vi "getMeasurement.vi"(7 "Source":string, 8 "error in (no error)":errorcluster, 10 "Measurement":T1=enum."Voltage Peak-Peak", 11 "ScopeKeysight in":refnum<class "ScopeKeysight.lvclass">) -> (0 "error out":errorcluster, 2 "Result":dbl, 3 "ScopeKeysight out":refnum<class "ScopeKeysight.lvclass">)   [LabVIEW 2023, in "ScopeKeysight.lvclass"]
doc: "<b>Author:</b> Wolfgang\n<b>Description:</b> returns a measurement"
uses:
  ScopeKeysight.lvclass
  Data/scopeMeasurements.ctl
  ScopeKeysight.lvclass/ScopeKeysight.ctl
  Driver/Public/Data/Read Measurement (Current Value).vi
  Driver/Keysight-DSQx3014T.lvlib
  sweScope.lvlib
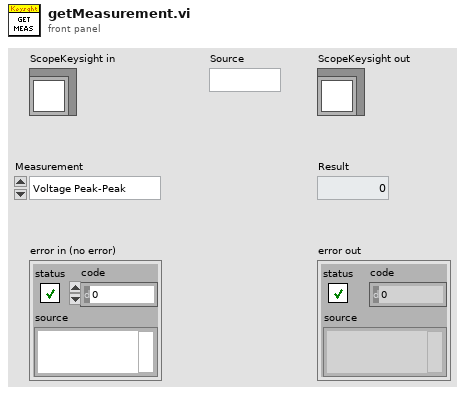
[diagram p1: front panel]
types:
  T1 = typedef "sweScope.lvlib/scopeMeasurements.ctl" = enum16{"Disable", "Mean", "Voltage Peak-Peak", "Frequency", "Amplitude", "Period", "Falling Slew Rate", "Rising Slew Rate"}
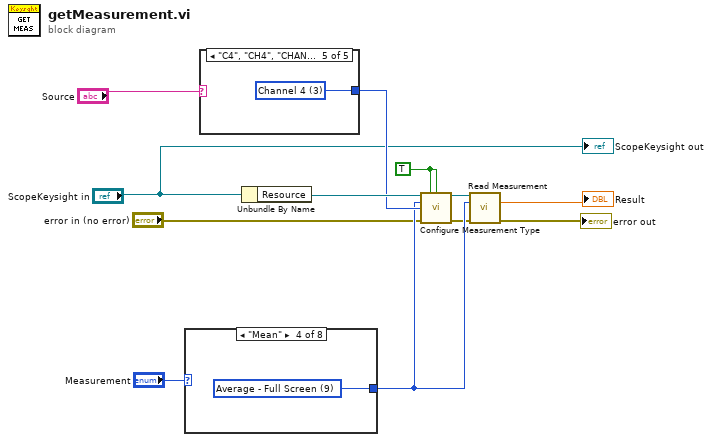
[diagram p0: block diagram]
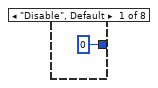
[diagram p2: hidden frame]
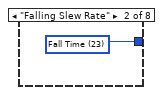
[diagram p3: hidden frame]
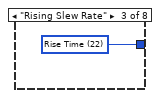
[diagram p4: hidden frame]
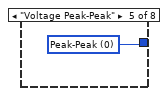
[diagram p5: hidden frame]
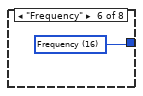
[diagram p6: hidden frame]
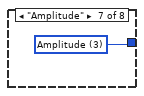
[diagram p7: hidden frame]
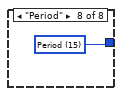
[diagram p8: hidden frame]
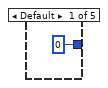
[diagram p9: hidden frame]
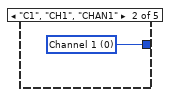
[diagram p10: hidden frame]
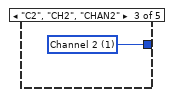
[diagram p11: hidden frame]
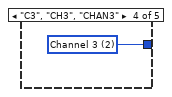
[diagram p12: hidden frame]
diagram:
  w1 = TRUE ("Enable Clear (F: Disable)")
  n1 = case shown="\"Mean\"" "Measurement" {
    tunnel: [0 ("Measurement Type (0: Peak-Peak)") w14 w15 w16 w17 w18 w19 w20] -> w8
    frame "Disable", Default {
    }
    frame "Falling Slew Rate" {
      w14 = 23 items=["Peak-Peak", "Maximum", "Mimimum", "Amplitude", "Top", "Base", "Overshoot", "Preshoot", "Average - N Cycles", "Average - Full Screen", "DC RMS - N Cycles", "DC RMS - Full Screen", "AC RMS - N Cycles", "AC RMS - Full Screen (Std Dev)", "Ratio", "Period", "Frequency", "Counter", "+Width", "-Width", "Burst Width", "Duty Cycle", "Rise Time", "Fall Time", "Delay", "Phase", "X minY", "X maxY", "Positive Pulse Count", "Negative Pulse Count", "Raising Edge Count", "Falling Edge Count", "Area - N Cycle", "Area - Full Screen", "Bit Rate", "Negtive Duty Cycle", "Standard Deviation"] ("Measurement Type (0: Peak-Peak)")
    }
    frame "Rising Slew Rate" {
      w15 = 22 items=["Peak-Peak", "Maximum", "Mimimum", "Amplitude", "Top", "Base", "Overshoot", "Preshoot", "Average - N Cycles", "Average - Full Screen", "DC RMS - N Cycles", "DC RMS - Full Screen", "AC RMS - N Cycles", "AC RMS - Full Screen (Std Dev)", "Ratio", "Period", "Frequency", "Counter", "+Width", "-Width", "Burst Width", "Duty Cycle", "Rise Time", "Fall Time", "Delay", "Phase", "X minY", "X maxY", "Positive Pulse Count", "Negative Pulse Count", "Raising Edge Count", "Falling Edge Count", "Area - N Cycle", "Area - Full Screen", "Bit Rate", "Negtive Duty Cycle", "Standard Deviation"] ("Measurement Type (0: Peak-Peak)")
    }
    frame "Mean" {
      w16 = 9 items=["Peak-Peak", "Maximum", "Mimimum", "Amplitude", "Top", "Base", "Overshoot", "Preshoot", "Average - N Cycles", "Average - Full Screen", "DC RMS - N Cycles", "DC RMS - Full Screen", "AC RMS - N Cycles", "AC RMS - Full Screen (Std Dev)", "Ratio", "Period", "Frequency", "Counter", "+Width", "-Width", "Burst Width", "Duty Cycle", "Rise Time", "Fall Time", "Delay", "Phase", "X minY", "X maxY", "Positive Pulse Count", "Negative Pulse Count", "Raising Edge Count", "Falling Edge Count", "Area - N Cycle", "Area - Full Screen", "Bit Rate", "Negtive Duty Cycle", "Standard Deviation"] ("Measurement Type (0: Peak-Peak)")
    }
    frame "Voltage Peak-Peak" {
      w17 = 0 items=["Peak-Peak", "Maximum", "Mimimum", "Amplitude", "Top", "Base", "Overshoot", "Preshoot", "Average - N Cycles", "Average - Full Screen", "DC RMS - N Cycles", "DC RMS - Full Screen", "AC RMS - N Cycles", "AC RMS - Full Screen (Std Dev)", "Ratio", "Period", "Frequency", "Counter", "+Width", "-Width", "Burst Width", "Duty Cycle", "Rise Time", "Fall Time", "Delay", "Phase", "X minY", "X maxY", "Positive Pulse Count", "Negative Pulse Count", "Raising Edge Count", "Falling Edge Count", "Area - N Cycle", "Area - Full Screen", "Bit Rate", "Negtive Duty Cycle", "Standard Deviation"] ("Measurement Type (0: Peak-Peak)")
    }
    frame "Frequency" {
      w18 = 16 items=["Peak-Peak", "Maximum", "Mimimum", "Amplitude", "Top", "Base", "Overshoot", "Preshoot", "Average - N Cycles", "Average - Full Screen", "DC RMS - N Cycles", "DC RMS - Full Screen", "AC RMS - N Cycles", "AC RMS - Full Screen (Std Dev)", "Ratio", "Period", "Frequency", "Counter", "+Width", "-Width", "Burst Width", "Duty Cycle", "Rise Time", "Fall Time", "Delay", "Phase", "X minY", "X maxY", "Positive Pulse Count", "Negative Pulse Count", "Raising Edge Count", "Falling Edge Count", "Area - N Cycle", "Area - Full Screen", "Bit Rate", "Negtive Duty Cycle", "Standard Deviation"] ("Measurement Type (0: Peak-Peak)")
    }
    frame "Amplitude" {
      w19 = 3 items=["Peak-Peak", "Maximum", "Mimimum", "Amplitude", "Top", "Base", "Overshoot", "Preshoot", "Average - N Cycles", "Average - Full Screen", "DC RMS - N Cycles", "DC RMS - Full Screen", "AC RMS - N Cycles", "AC RMS - Full Screen (Std Dev)", "Ratio", "Period", "Frequency", "Counter", "+Width", "-Width", "Burst Width", "Duty Cycle", "Rise Time", "Fall Time", "Delay", "Phase", "X minY", "X maxY", "Positive Pulse Count", "Negative Pulse Count", "Raising Edge Count", "Falling Edge Count", "Area - N Cycle", "Area - Full Screen", "Bit Rate", "Negtive Duty Cycle", "Standard Deviation"] ("Measurement Type (0: Peak-Peak)")
    }
    frame "Period" {
      w20 = 15 items=["Peak-Peak", "Maximum", "Mimimum", "Amplitude", "Top", "Base", "Overshoot", "Preshoot", "Average - N Cycles", "Average - Full Screen", "DC RMS - N Cycles", "DC RMS - Full Screen", "AC RMS - N Cycles", "AC RMS - Full Screen (Std Dev)", "Ratio", "Period", "Frequency", "Counter", "+Width", "-Width", "Burst Width", "Duty Cycle", "Rise Time", "Fall Time", "Delay", "Phase", "X minY", "X maxY", "Positive Pulse Count", "Negative Pulse Count", "Raising Edge Count", "Falling Edge Count", "Area - N Cycle", "Area - Full Screen", "Bit Rate", "Negtive Duty Cycle", "Standard Deviation"] ("Measurement Type (0: Peak-Peak)")
    }
  }
  n2 = case shown="\"C4\", \"CH4\", \"CHAN4\"" "Source" {
    tunnel: [0 ("Channel Name (0: Channel 1)") w22 w23 w24 w25] -> w9
    frame Default {
    }
    frame "C1", "CH1", "CHAN1" {
      w22 = 0 items=["Channel 1", "Channel 2", "Channel 3", "Channel 4"] ("Channel Name (0: Channel 1)")
    }
    frame "C2", "CH2", "CHAN2" {
      w23 = 1 items=["Channel 1", "Channel 2", "Channel 3", "Channel 4"] ("Channel Name (0: Channel 1)")
    }
    frame "C3", "CH3", "CHAN3" {
      w24 = 2 items=["Channel 1", "Channel 2", "Channel 3", "Channel 4"] ("Channel Name (0: Channel 1)")
    }
    frame "C4", "CH4", "CHAN4" {
      w25 = 3 items=["Channel 1", "Channel 2", "Channel 3", "Channel 4"] ("Channel Name (0: Channel 1)")
    }
  }
  n3 = Unbundle By Name("ScopeKeysight in") -> ("Resource"=w11:refnum<visa-resource-name>)
  n4 = call "Configure Measurement Type.vi"("VISA resource name"=w11, "Enable Clear (F: Disable)"=w1, "Enable Statistics Reset (F: Disable)"=w1, "Measurement Type (0: Peak-Peak)"=w8, "Measurement Source 1 (0: Channel 1)"=w9, "error in (no error)"="error in (no error)") -> ("VISA resource name out"=w10:refnum<visa-resource-name>, "error out"=w6:errorcluster)  [unwired: 8 in]
  n5 = call-poly "Read Measurement.vi"("VISA resource name"=w10, "Measurement Type (0: Peak-Peak)"=w8, "error in (no error)"=w6) -> ("Result Value"=→"Result":dbl, "error out"=→"error out":errorcluster)  [unwired: 10 in, 1 out]
  "ScopeKeysight out" <- "ScopeKeysight in"
